vi "write progress dialog.vi"() -> ()   [LabVIEW 2018]
uses:
  CAEN globals.vi
panel:
  out "Message":string="Setting crate... \r\nSetting screen...\r\nSetting group... \r\nSetting page... \r\nSetting subpage...\r\nSetting row... \r\nSetting column... \r\nWriting value... \r\n"
  out "Writing...":u8(slide) scale=0.0..100.0
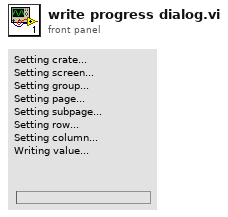
[diagram p1: front panel]
types:
  T1 = enum32{"Invalid", "Standard", "Closed", "Hidden", "Minimized", "Maximized"}
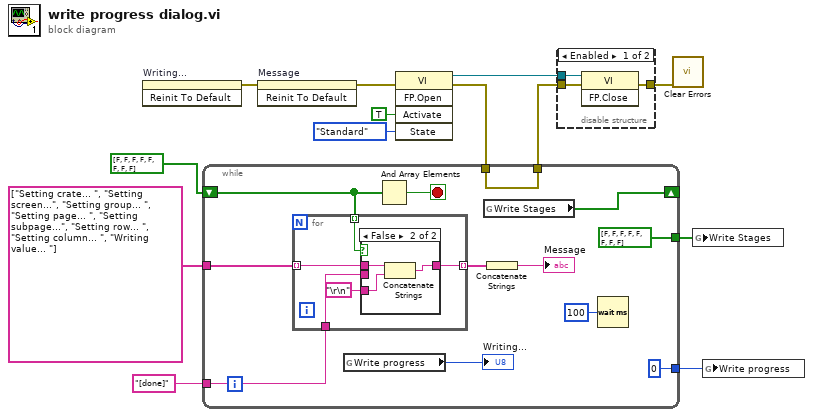
[diagram p0: block diagram]
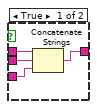
[diagram p3: hidden frame]
diagram:
  n1 = invoke on="Writing..." class="Slide (strict)" method="Reinit To Default"() -> (error out=w2:errorcluster)  [unwired: 3 in, 2 out]
  n2 = invoke on="Message" class="Str" method="Reinit To Default"(error in=w2) -> (error out=w3:errorcluster)  [unwired: 2 in, 2 out]
  n3 = invoke class="VI" method="FP.Open"(error in=w3, "Activate"=TRUE ("Activate?"), "State"=T1."Standard") -> (reference out=w6:refnum<vi>, error out=w11:errorcluster)  [unwired: 2 in, 3 out]
  n4 = while {
    tunnel: string[] ["Setting crate... ", "Setting screen...", "Setting group... ", "Setting page... ", "Setting subpage...", "Setting row... ", "Setting column... ", "Writing value... "] ("array 2") -> [w25]
    tunnel: "[done]" ("Message") -> [w24]
    tunnel: [u8 0 ("milliseconds to wait")] -> w13
    tunnel: [bool[] [FALSE, FALSE, FALSE, FALSE, FALSE, FALSE, FALSE, FALSE] ("Write Stages")] -> w12
    tunnel: [w16] -> w5
    tunnel: w11 -> [w16]
    shift-right: [w15] -> _
    shift-left: bool[] [FALSE, FALSE, FALSE, FALSE, FALSE, FALSE, FALSE, FALSE] ("Write Stages") -> [w14]
    stop <- w21 stop-if-true
    n5 = for {
      tunnel: w25 -> [w30] mode=indexing
      tunnel: w24 -> [w29]
      tunnel: [w28] -> w23 mode=indexing
      tunnel: w14 -> [w26] mode=indexing
      n6 = case shown="False" w26 {
        tunnel: w30 -> [w34 w37]
        tunnel: w29 -> [w33 _]
        tunnel: [w32 w36] -> w28
        tunnel: "\r\n" -> [w31 w35]
        frame True {
          n7 = Concatenate Strings(w34, w33, w31) -> (w32:string)
        }
        frame False {
          n8 = Concatenate Strings(w37, w35) -> (w36:string)
        }
      }
    }
    n9 = global read "CAEN globals.vi" "Write progress"() -> (→"Writing...":u8)
    n10 = And Array Elements(Boolean array=w14) -> (logical AND=w21:bool)
    n11 = global read "CAEN globals.vi" "Write Stages"() -> (w15:bool[])
    n12 = Concatenate Strings(w23) -> (→"Message":string)
    n13 = Wait (ms)(milliseconds to wait=u32 100) -> ()  [unwired: 1 out]
  }
  n14 = disable-structure shown="Enabled" {
    disable-tunnel: w6 -> [w40 _]
    disable-tunnel: w5 -> [w39 w41]
    disable-tunnel: [w38 w41] -> w4
    frame Enabled {
      n15 = invoke class="VI" method="FP.Close"(reference=w40, error in=w39) -> (error out=w38:errorcluster)  [unwired: 1 in, 2 out]
    }
    frame Disabled {
    }
  }
  n16 = call <vilib>:"Clear Errors.vi"("error in (no error)"=w4) -> ()  [unwired: 5 in, 2 out]
  n17 = global write "CAEN globals.vi" "Write Stages"(w12) -> ()
  n18 = global write "CAEN globals.vi" "Write progress"(w13) -> ()
